vi "ProgramBitstreamWriteMeasurementFileReadCurrent.vi"() -> ()   [LabVIEW 2009]
panel:
  in  "file path (use dialog) 2":path
  in  "file path (use dialog)":path
  out "return code":i32
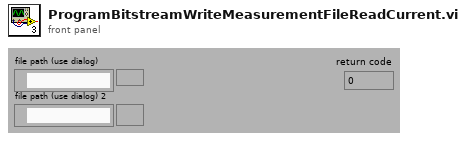
[diagram p1: front panel]
types:
  T1 = enum16{"open", "replace", "create", "open or create", "replace or create", "replace or create with confirmation"}
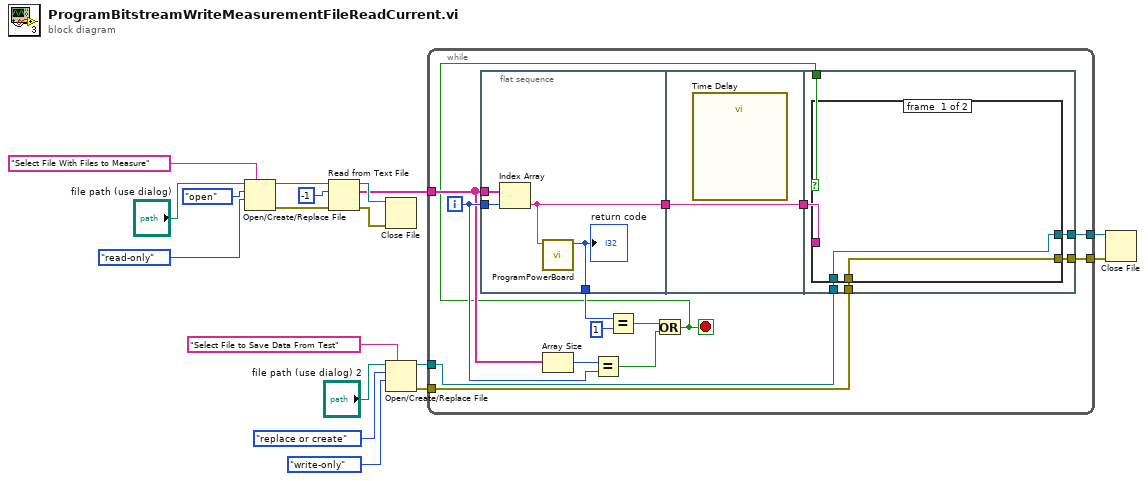
[diagram p0: block diagram]
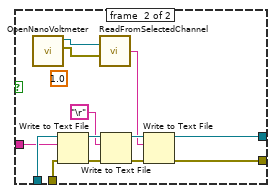
[diagram p2: hidden frame]
diagram:
  n1 = Open/Create/Replace File(file path (use dialog)="file path (use dialog)", prompt="Select File With Files to Measure", operation (0:open)=T1."open", access (0:read/write)=enum16{"read/write", "read-only", "write-only"}."read-only") -> (refnum out=w14:refnum<file>, error out=w11:errorcluster)  [unwired: 2 in, 1 out]
  n2 = Read from Text File(file (use dialog)=w14, count=-1, error in=w11) -> (refnum out=w13:refnum<file>, text=w5:string[], error out=w12:errorcluster)  [unwired: 1 in, 1 out]
  n3 = Close File(refnum=w13, error in=w12) -> ()  [unwired: 2 out]
  n4 = Open/Create/Replace File(file path (use dialog)="file path (use dialog) 2", prompt="Select File to Save Data From Test", operation (0:open)=T1."replace or create", access (0:read/write)=enum16{"read/write", "read-only", "write-only"}."write-only") -> (refnum out=w4:refnum<file>, error out=w1:errorcluster)  [unwired: 2 in, 1 out]
  n5 = while {
    tunnel: w5 -> [w27]
    tunnel: w4 -> [w25]
    tunnel: [w24] -> w3
    tunnel: [w23] -> w2
    tunnel: w1 -> [w22]
    i -> [w28]
    stop <- w19 stop-if-true
    n6 = flat-sequence {
      tunnel: [w36] -> w31
      tunnel: w27 -> [w34]
      tunnel: w28 -> [w35]
      tunnel: [w33] -> w21
      tunnel: w21 -> [w37]
      tunnel: [w37] -> w20
      tunnel: w20 -> [w39]
      tunnel: w25 -> [w41]
      tunnel: [w43] -> w24
      tunnel: [w42] -> w23
      tunnel: w22 -> [w40]
      tunnel: w19 -> [w38]
      frame #0 {
        n7 = Index Array(array=w34, index=w35) -> (element=w33:string)
        n8 = call "ProgramPowerBoard.vi"("BitstreamFilename"=w33) -> ("return code"=w36:i32)  [unwired: 10 in]
        "return code" <- w36
      }
      frame #1 {
        n9 = call "Time Delay"() -> ()  [unwired: 11 in, 1 out]
      }
      frame #2 {
        n10 = case shown="False" w38 {
          tunnel: [w44 w50] -> w43
          tunnel: [w45 w49] -> w42
          tunnel: w41 -> [w44 w54]
          tunnel: w40 -> [w45 w53]
          tunnel: w39 -> [_ w52]
          frame #0 {
          }
          frame #1 {
            (unwired) 1.0 ("ChannelSelection")
            n11 = call "OpenNanoVoltmeter.vi"() -> ("error out"=w47:errorcluster, "reference out"=w48:refnum<visa-resource-name>)  [unwired: 8 in]
            n12 = Write to Text File(file (use dialog)=w54, text=w52, error in=w53) -> (refnum out=w55:refnum<file>, error out=w56:errorcluster)  [unwired: 1 in, 1 out]
            n13 = call "ReadFromSelectedChannel.vi"("reference out 3"=w48, "error out"=w47) -> ("read buffer"=w46:string)  [unwired: 2 out]
            n14 = Write to Text File(file (use dialog)=w55, text="\r", error in=w56) -> (refnum out=w58:refnum<file>, error out=w57:errorcluster)  [unwired: 1 in, 1 out]
            n15 = Write to Text File(file (use dialog)=w58, text=w46, error in=w57) -> (refnum out=w50:refnum<file>, error out=w49:errorcluster)  [unwired: 1 in, 1 out]
          }
        }
      }
    }
    n16 = Array Size(array=w27) -> (size(s)=w26:i32)
    n17 = Equal?(x=w26, y=w28) -> (x = y?=w32:bool)
    n18 = Equal?(x=w31, y=1) -> (x = y?=w29:bool)
    n19 = Or(x=w29, y=w32) -> (x .or. y?=w19:bool)
  }
  n20 = Close File(refnum=w3, error in=w2) -> ()  [unwired: 2 out]
